vi "ADAM Control ALL Relays.vi"() -> ()   [LabVIEW 2014]
panel:
  in  "State":bool
  in  "ADAM IP Address":string="127.0.0.1"
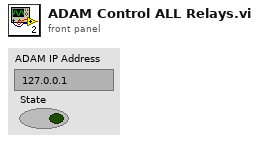
[diagram p1: front panel]
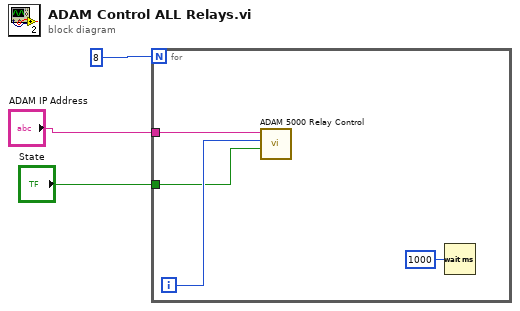
[diagram p0: block diagram]
diagram:
  n1 = for {
    N: 8 ("Numeric") -> [_]
    tunnel: "ADAM IP Address" -> [w6]
    tunnel: "State" -> [w5]
    i -> [w7]
    n2 = call "ADAM 5000 Relay Control.vi"("State"=w5, "Relay #"=w7, "Remote IP Address 2"=w6) -> ()  [unwired: 9 in]
    n3 = Wait (ms)(milliseconds to wait=u32 1000) -> ()  [unwired: 1 out]
  }
